vi "2100_SP3T_Meas and Cal_Resitance.vi"(0 "Instrument Sessions":refnum<k15>[](array[refnum]), 1 "Current  Level":dbl=-1e-05 format="%#_6p", 5 "Channel Lists":string[](array[string]), 11 "error in (no error)":errorcluster) -> (4 "Instrument Sessions out":refnum<k15>[](array[refnum]), 6 "Channel Lists Out":string[](array[string]), 8 "Individual_Resitances":dbl[](array[numeric]), 10 "Parallel_Resitance":dbl[](array[numeric]), 15 "error out":errorcluster)   [LabVIEW 2013]
uses:
  <instrlib>/niDCPower/nidcpower.llb/niDCPower Wait For Event - Event.ctl
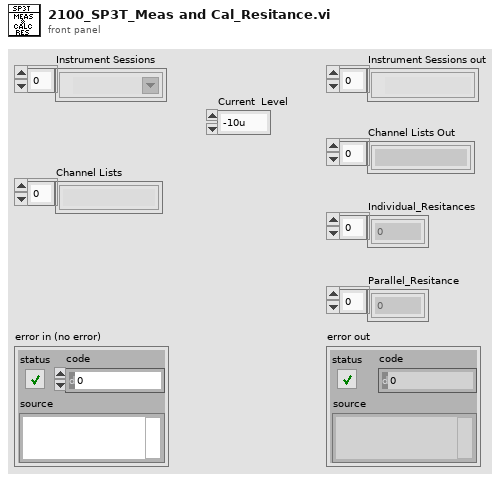
[diagram p1: front panel]
types:
  T1 = typedef "niDCPower Wait For Event - Event.ctl" = i32
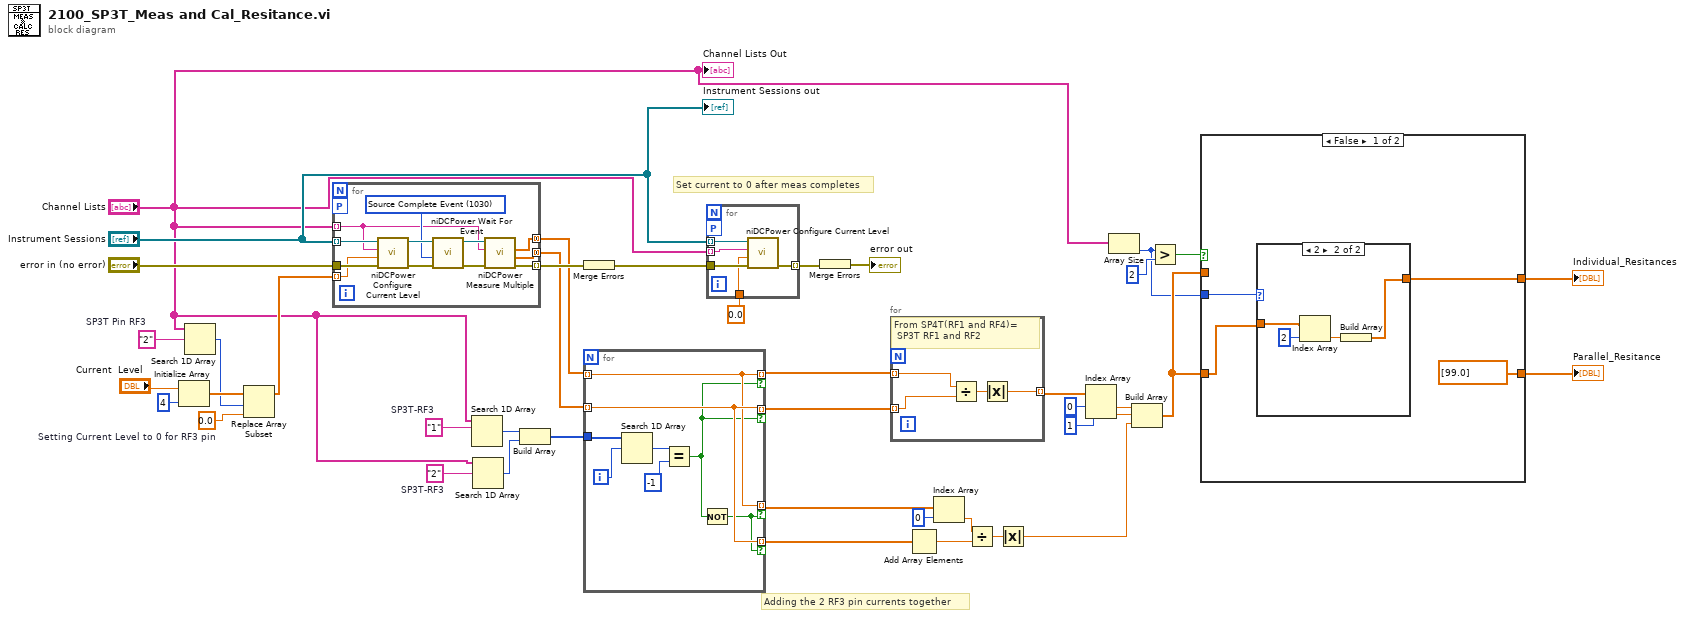
[diagram p0: block diagram]
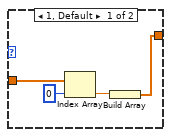
[diagram p2: hidden frame]
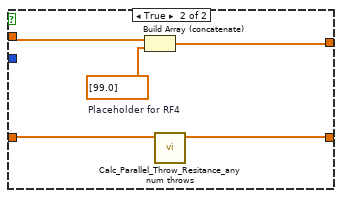
[diagram p3: hidden frame]
diagram:
  w8 = "2"  # SP3T Pin RF3
  w31 = "2"  # SP3T-RF3
  w32 = "1"  # SP3T-RF3
  w39 = 0.0  # Setting Current Level to 0 for RF3 pin
  # "Set current to 0 after meas completes"
  # "Adding the 2 RF3 pin currents together"
  n1 = Initialize Array("Current  Level", 4 ("dimension size")) -> (w40:dbl[])
  n2 = Search 1D Array(1D array="Channel Lists", element=w8) -> (index of element=w33:i32)  [unwired: 1 in]
  n3 = Replace Array Subset(array=w40, new element=w39, index=w33) -> (w34:dbl[])
  n4 = for {
    tunnel: "error in (no error)" -> [w49]
    tunnel: "Instrument Sessions" -> [w48] mode=indexing
    tunnel: [w47] -> w37 mode=indexing
    tunnel: "Channel Lists" -> [w45] mode=indexing
    tunnel: w34 -> [w46] mode=indexing
    workers-P: _ -> [_]
    tunnel: [w44] -> w27 mode=concatenating
    tunnel: [w43] -> w28 mode=concatenating
    w51 = T1 1030 items=["Source Complete Event"=1030, "Measure Complete Event"=1031, "Sequence Iteration Complete Event"=1032, "Sequence Engine Done Event"=1033, "Pulse Complete Event"=1051, "Ready For Pulse Trigger Event"=1052] ("event")
    n5 = call <instrlib>:"niDCPower Configure Current Level.vi"("error in (no error)"=w49, "current level"=w46, "channel name"=w45, "instrument handle"=w48) -> ("error out"=w50:errorcluster, "instrument handle out"=w52:refnum<k15>)  [unwired: 6 in]
    n6 = call <instrlib>:"niDCPower Wait For Event.vi"("error in (no error)"=w50, "event"=w51, "instrument handle"=w52) -> ("error out"=w53:errorcluster, "instrument handle out"=w54:refnum<k15>)  [unwired: 7 in]
    n7 = call <instrlib>:"niDCPower Measure Multiple.vi"("error in (no error)"=w53, "channel name"=w45, "instrument handle"=w54) -> ("error out"=w47:errorcluster, "current measurements"=w43:dbl[], "voltage measurements"=w44:dbl[])  [unwired: 5 in, 1 out]
  }
  n8 = Search 1D Array(1D array="Channel Lists", element=w32) -> (index of element=w22:i32)  [unwired: 1 in]
  n9 = Search 1D Array(1D array="Channel Lists", element=w31) -> (index of element=w30:i32)  [unwired: 1 in]
  n10 = Build Array(w22, w30) -> (w29:i32[])
  n11 = Merge Errors(w37) -> (w38:errorcluster)
  n12 = for {
    tunnel: w29 -> [w62]
    tunnel: w28 -> [w58] mode=indexing
    tunnel: w27 -> [w57] mode=indexing
    tunnel: [w58] -> w25 mode=indexing if=w56
    tunnel: [w57] -> w26 mode=indexing if=w56
    tunnel: [w58] -> w24 mode=indexing if=w55
    tunnel: [w57] -> w23 mode=indexing if=w55
    i -> [w61]
    n13 = Search 1D Array(1D array=w62, element=w61) -> (index of element=w60:i32)  [unwired: 1 in]
    n14 = Equal?(x=w60, y=-1) -> (x = y?=w56:bool)
    n15 = Not(x=w56) -> (.not. x?=w55:bool)
  }
  n16 = for {
    tunnel: w38 -> [w67]
    tunnel: [w66] -> w36 mode=indexing
    tunnel: "Instrument Sessions" -> [w65] mode=indexing
    tunnel: "Channel Lists" -> [w64] mode=indexing
    tunnel: 0.0 ("current level") -> [w63]
    workers-P: _ -> [_]
    n17 = call <instrlib>:"niDCPower Configure Current Level.vi"("error in (no error)"=w67, "current level"=w63, "channel name"=w64, "instrument handle"=w65) -> ("error out"=w66:errorcluster)  [unwired: 6 in, 1 out]
  }
  n18 = Merge Errors(w36) -> (→"error out":errorcluster)
  n19 = for {
    tunnel: w26 -> [w70] mode=indexing
    tunnel: w25 -> [w69] mode=indexing
    tunnel: [w68] -> w18 mode=indexing
    # "From SP4T(RF1 and RF4)=\n SP3T RF1 and RF2"
    n20 = Divide(x=w70, y=w69) -> (x/y=w71:dbl)
    n21 = Absolute Value(x=w71) -> (abs(x)=w68:dbl)
  }
  n22 = Add Array Elements(numeric array=w24) -> (sum=w19:dbl)
  n23 = Index Array(array=w23, index=0) -> (element=w20:dbl)
  n24 = Divide(x=w20, y=w19) -> (x/y=w21:dbl)
  n25 = Absolute Value(x=w21) -> (abs(x)=w13:dbl)
  n26 = Index Array(array=w18, index #1=0 ("index"), index #2=1 ("index")) -> (element #1=w15:dbl, element #2=w14:dbl)
  n27 = Array Size(array="Channel Lists") -> (size(s)=w1:i32)
  n28 = Build Array(w15, w14, w13) -> (w3:dbl[])
  n29 = Greater?(x=w1, y=2) -> (0:w6:bool)
  n30 = case shown="False" w6 {
    tunnel: w3 -> [_ w87]
    tunnel: [w72 w85] -> w4
    tunnel: w3 -> [w73 w86]
    tunnel: [dbl[] [99.0] ("Parallel_Resitance") w84] -> w2
    tunnel: w1 -> [w74 _]
    frame False {
      n31 = case shown="2" w74 {
        tunnel: w73 -> [w79 w83]
        tunnel: [w76 w80] -> w72
        frame 1, Default {
          n32 = Index Array(array=w79, index=0) -> (element=w77:dbl)
          n33 = Build Array(w77) -> (w76:dbl[])
        }
        frame 2 {
          n34 = Index Array(array=w83, index=2) -> (element=w81:dbl)
          n35 = Build Array(w81) -> (w80:dbl[])
        }
      }
    }
    frame True {
      w88 = dbl[] [99.0]  # Placeholder for RF4
      n36 = Build Array (concatenate)(w87, w88) -> (w85:dbl[])
      n37 = call "Calc_Parallel_Throw_Resitance_any num throws.vi"("Resitance_Per Site"=w86) -> ("Parallel_Resitance"=w84:dbl[])  [unwired: 10 in]
    }
  }
  "Individual_Resitances" <- w4
  "Parallel_Resitance" <- w2
  "Instrument Sessions out" <- "Instrument Sessions"
  "Channel Lists Out" <- "Channel Lists"
